vi "process file converter.vi"() -> ()   [LabVIEW 2021]
uses:
  NHMFL_Core/Libraries/File/File Format Converter/Format Converter Configuration.ctl
panel:
  in  "Configuration":T1={"New start time"=nan, "New end time"=nan, "Output file format"=enum."ASCII", "Save ASCII column names"=TRUE, "Prepend binary array size"=FALSE, "buffer size (-1: all)"=100000, "Channels"=["jsdhgv", "lsjdfh", "ajlsd"], "Group"="p", "New dt"=nan} {"buffer size (-1: all)" format="%.0p"; "New start time" format="%#_10p"}
  in  "Folder Path":path=path "/opt/Dropbox/shared_Ali/nanocal-March2020 - RuCl3/March_2020"
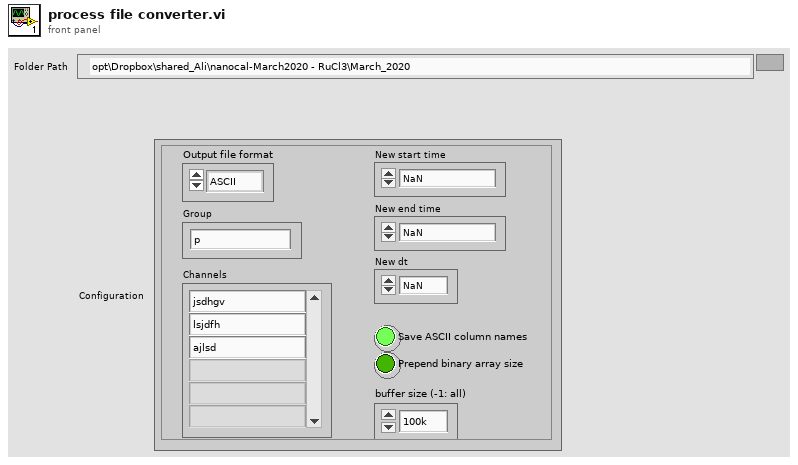
[diagram p1: front panel]
types:
  T1 = typedef "Format Converter Configuration.ctl" = cluster{"New start time":dbl, "New end time":dbl, "Output file format":enum16{"ASCII", "BINARY", "TDMS"}, "Save ASCII column names":bool, "Prepend binary array size":bool, "buffer size (-1: all)":i64, "Channels":string[], "Group":string, "New dt":dbl}
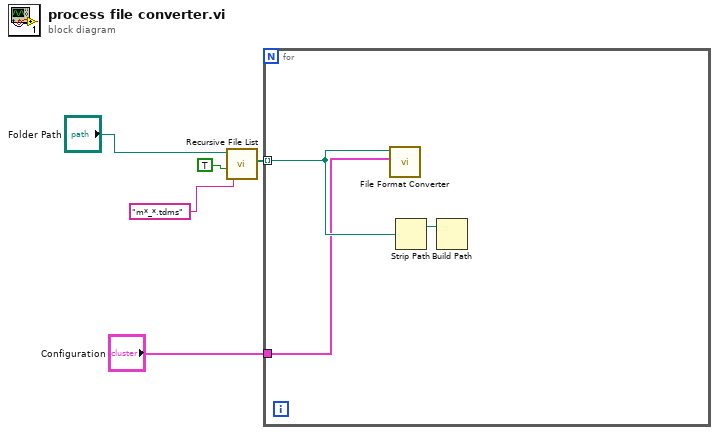
[diagram p0: block diagram]
diagram:
  n1 = call <vilib>:"Recursive File List.vi"("pattern"="m*_*.tdms", "Continue Recursing on Error? (F)"=TRUE, "Folder Path"="Folder Path") -> ("All Files in Dir"=w2:path[])  [unwired: 4 in, 4 out]
  n2 = for {
    tunnel: w2 -> [w8] mode=indexing
    tunnel: "Configuration" -> [w6]
    n3 = call "File Format Converter.vi"("Configuration"=w6, "File"=w8) -> ()  [unwired: 7 in, 3 out]
    n4 = Strip Path(path=w8) -> (stripped path=w7:path)  [unwired: 1 out]
    n5 = Build Path(base path=w7) -> ()  [unwired: 1 in, 1 out]
  }
